vi "Invoke Method.vi"(8 "error in (no error)":errorcluster, 9 "In Parameters":variant[](array[variant]), 10 "Function Block#Method":string, 11 "TwinCAT ADS in":refnum<class "TwinCAT ADS.lvclass">) -> (0 "error out":errorcluster, 1 "Out Parameters":variant[](array[variant]), 2 "Return":variant, 3 "TwinCAT ADS out":refnum<class "TwinCAT ADS.lvclass">)   [LabVIEW 2018, in "TwinCAT ADS.lvclass"]
uses:
  TwinCAT ADS.lvclass
  TwinCAT ADS.lvclass/TwinCAT ADS.ctl
  TwinCAT.Ads
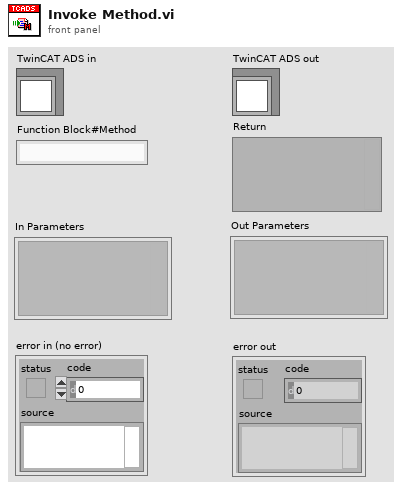
[diagram p1: front panel]
types:
  T1 = typedef "TwinCAT ADS.lvclass/PLC RPC Type Descriptor.ctl" = cluster{"Return Type Name":string, "Return Type Byte Size":i32, "In Parameters":T2[], "Out Parameters":T2[]}
  T2 = typedef "TwinCAT ADS.lvclass/PLC RPC Parameter Type Descriptor.ctl" = cluster{"Type Name":string, "Size":i32}
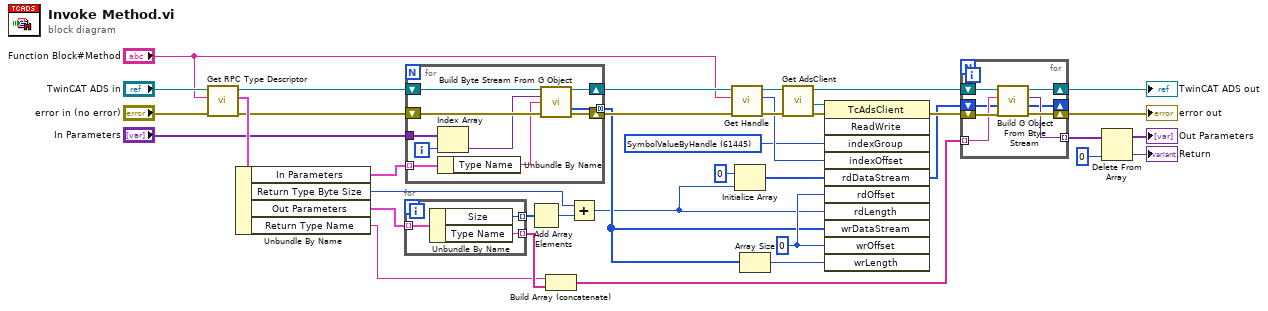
[diagram p0: block diagram]
diagram:
  w22 = 0 ("wrOffset")
  w35 = u32 61445 items=["PlcRWIB"=16384, "PlcRWOB"=16400, "PlcRWMB"=16416, "PlcRWRB"=16432, "PlcRWDB"=16448, "SymbolTable"=61440, "SymbolName"=61441, "SymbolValue"=61442, "SymbolHandleByName"=61443, "SymbolValueByName"=61444, "SymbolValueByHandle"=61445, "SymbolReleaseHandle"=61446, "SymbolInfoByName"=61447, "SymbolVersion"=61448, "SymbolInfoByNameEx"=61449, "SymbolDownload"=61450, "SymbolUpload"=61451, "SymbolUploadInfo"=61452, "SymbolNote"=61456, "IOImageRWIB"=61472, "IOImageRWIX"=61473, "IOImageRWOB"=61488, "IOImageRWOX"=61489, "IOImageClearI"=61504, "IOImageClearO"=61520, "SumCommandRead"=61568, "SumCommandWrite"=61569, "SumCommandReadWrite"=61570, "SumCommandReadEx"=61571, "SumCommandReadEx2"=61572, "SumCommandAddDevNote"=61573, "SumCommandDelDevNote"=61574, "DeviceData"=61696] ("SumCommandRead")
  n1 = call "Get RPC Type Descriptor.vi"("error in (no error)"="error in (no error)", "Function Block#Method"="Function Block#Method", "TwinCAT ADS in"="TwinCAT ADS in") -> ("error out"=w28:errorcluster, "RPC Type Descriptor"=w32:T1, "TwinCAT ADS out"=w29:refnum<class "TwinCAT ADS.lvclass">)  [unwired: 6 in]
  n2 = Unbundle By Name(w32) -> ("In Parameters"=w27:T2[], "Return Type Byte Size"=w16:i32, "Out Parameters"=w19:T2[], "Return Type Name"=w13:string)
  n3 = for {
    tunnel: w19 -> [w41] mode=indexing
    tunnel: [w40] -> w18 mode=indexing
    tunnel: [w39] -> w14 mode=indexing
    n4 = Unbundle By Name(w41) -> ("Size"=w40:i32, "Type Name"=w39:string)
  }
  n5 = for {
    shift-right: [w47] -> w23
    shift-left: w29 -> [w51]
    shift-right: [w46] -> w25
    shift-left: w28 -> [w49]
    tunnel: w27 -> [w50] mode=indexing
    tunnel: "In Parameters" -> [w45]
    tunnel: [w42] -> w21 mode=concatenating
    i -> [w44]
    n6 = Index Array(array=w45, index=w44) -> (element=w43:variant)
    n7 = Unbundle By Name(w50) -> ("Type Name"=w48:string)
    n8 = call "Build Byte Stream From G Object.vi"("TwinCAT ADS in"=w51, "Value"=w43, "Type Name"=w48, "error in (no error)"=w49) -> ("TwinCAT ADS out"=w47:refnum<class "TwinCAT ADS.lvclass">, "Byte Stream out"=w42:u8[], "error out"=w46:errorcluster)  [unwired: 9 in]
  }
  n9 = Add Array Elements(numeric array=w18) -> (sum=w17:i32)
  n10 = Build Array (concatenate)(w13, w14) -> (w12:string[])
  n11 = Add(x=w16, y=w17) -> (x+y=w15:i32)
  n12 = call "Get Handle.vi"("error in (no error)"=w25, "Symbol Name"="Function Block#Method", "TwinCAT ADS in"=w23) -> ("error out"=w38:errorcluster, "Handle"=w36:i32, "TwinCAT ADS out"=w37:refnum<class "TwinCAT ADS.lvclass">)  [unwired: 6 in]
  n13 = Initialize Array(u8 0, w15) -> (w24:u8[])
  n14 = Array Size(array=w21) -> (size(s)=w20:i32)
  n15 = call "Get AdsClient.vi"("error in (no error)"=w38, "TwinCAT ADS in"=w37) -> ("error out"=w34:errorcluster, ".NET TcAdsClient"=w33:refnum<k24>, "TwinCAT ADS out"=w30:refnum<class "TwinCAT ADS.lvclass">)  [unwired: 7 in]
  n16 = invoke class="TcAdsClient" method="ReadWrite"(reference=w33, error in=w34, "indexGroup"=w35, "indexOffset"=w36, "rdDataStream"=w24, "rdOffset"=w22, "rdLength"=w15, "wrDataStream"=w21, "wrOffset"=w22, "wrLength"=w20) -> (error out=w31:errorcluster, "rdDataStream"=w1:u8[])  [unwired: 1 in, 9 out]
  n17 = for {
    shift-right: [w58] -> w5
    shift-left: w31 -> [w57]
    shift-right: [w59] -> w4
    shift-left: w30 -> [w56]
    shift-right: [w53] -> _
    shift-left: w1 -> [w52]
    tunnel: w12 -> [w54] mode=indexing
    tunnel: [w55] -> w10 mode=indexing
    n18 = call "Build G Object From Btye Stream.vi"("error in (no error)"=w57, "Byte Stream in"=w52, "Type Name"=w54, "TwinCAT ADS in"=w56) -> ("error out"=w58:errorcluster, "Byte Stream out"=w53:u8[], "Value"=w55:variant, "TwinCAT ADS out"=w59:refnum<class "TwinCAT ADS.lvclass">)  [unwired: 4 in]
  }
  "error out" <- w5
  "TwinCAT ADS out" <- w4
  n19 = Delete From Array(array=w10, index=0) -> (deleted portion=→"Return":variant, array with subset deleted=→"Out Parameters":variant[])  [unwired: 1 in]
